vi "Case Structure SB.vi"() -> ()   [LabVIEW 2019]
panel:
  in  "String":string
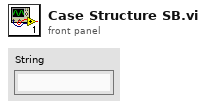
[diagram p1: front panel]
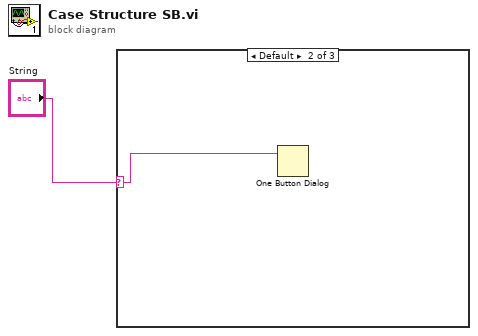
[diagram p0: block diagram]
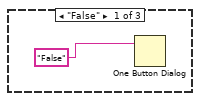
[diagram p2: hidden frame]
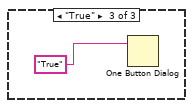
[diagram p3: hidden frame]
diagram:
  n1 = case shown="Default" "String" {
    selector: "String" -> [_ w3 _]
    frame "False" {
      n2 = One Button Dialog(message="False") -> ()  [unwired: 1 in, 1 out]
    }
    frame Default {
      n3 = One Button Dialog(message=w3) -> ()  [unwired: 1 in, 1 out]
    }
    frame "True" {
      n4 = One Button Dialog(message="True") -> ()  [unwired: 1 in, 1 out]
    }
  }
